vi "Webcam_Image2String.vi"(7 "file (use dialog)":path=path "/home/pi/temp.jpg", 8 "error in (no error)":errorcluster, 10 "imagegray":u8[][](array[numeric]), 11 "Image Pixels":u32[][](array[numeric])) -> (0 "error out":errorcluster, 3 "string":string)   [LabVIEW 2014, in "QwaveSys RPi Training Library.lvlib"]
uses:
  <vilib>/Q-Wave Systems/QwaveSys RPi Training Package (Demo)/Addons/QwaveSys RPi Training Library.lvlib
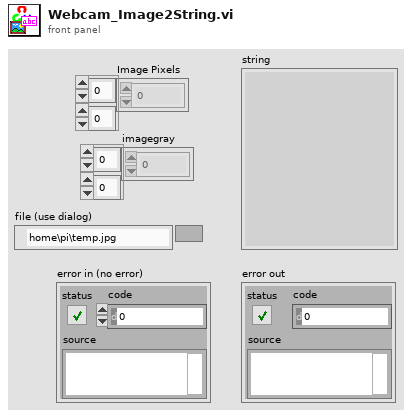
[diagram p1: front panel]
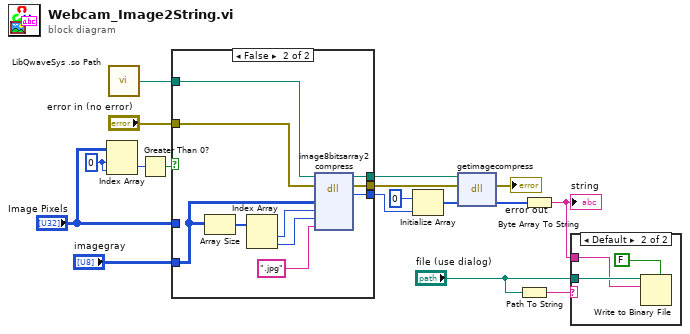
[diagram p0: block diagram]
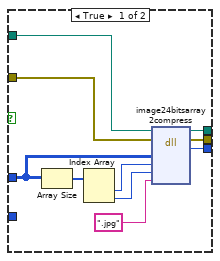
[diagram p2: hidden frame]
diagram:
  w6 = 0 ("index (row)")
  n1 = Index Array(array="Image Pixels", index (row)=w6, index (col)=w6) -> (element=w4:u32)
  n2 = call <vilib>:"LibQwaveSys .so Path.vi"() -> ("Lib QwaveSys .so Path"=w3:path)  [unwired: 5 in]
  n3 = Greater Than 0?(x=w4) -> (x > 0?=w5:bool)
  n4 = case shown="False" w5 {
    tunnel: [w27 w37] -> w15
    tunnel: [w26 w36] -> w14
    tunnel: "Image Pixels" -> [w21 _]
    tunnel: "imagegray" -> [_ w31]
    tunnel: w3 -> [w20 w30]
    tunnel: "error in (no error)" -> [w18 w29]
    tunnel: [w19 w28] -> w1
    frame True {
      n5 = Array Size(array=w21) -> (size(s)=w25:i32[])
      n6 = Index Array(array=w25) -> (element #1=w22:i32, element #2=w23:i32)  [unwired: 2 in]
      n7 = dll-call lib="libqwavesys.so" fn="image24bitsarray2compress"(path in=w20, error in=w18, "img"=w21, "cols"=w22, "rows"=w23, "file_extension"=".jpg") -> (path out=w19:path, error out=w27:errorcluster, "return type"=w26:i32)  [unwired: 5 in]
    }
    frame False {
      n8 = Array Size(array=w31) -> (size(s)=w35:i32[])
      n9 = Index Array(array=w35) -> (element #1=w32:i32, element #2=w33:i32)  [unwired: 2 in]
      n10 = dll-call lib="libqwavesys.so" fn="image8bitsarray2compress"(path in=w30, error in=w29, "img"=w31, "cols"=w32, "rows"=w33, "file_extension"=".jpg") -> (path out=w28:path, error out=w37:errorcluster, "return type"=w36:i32)  [unwired: 5 in]
    }
  }
  n11 = Initialize Array(u8 0 ("data"), w14) -> (w12:u8[])
  n12 = dll-call lib="libqwavesys.so" fn="getimagecompress"(path in=w1, error in=w15, "data"=w12) -> (error out=→"error out":errorcluster, "data"=w16:u8[])  [unwired: 2 in, 1 out]
  n13 = Path To String(path="file (use dialog)") -> (string=w10:string)
  n14 = Byte Array To String(unsigned byte array=w16) -> (string=w13:string)
  "string" <- w13
  n15 = case shown="Default" w10 {
    tunnel: "file (use dialog)" -> [_ w39]
    tunnel: w13 -> [_ w38]
    frame "/" {
    }
    frame Default {
      n16 = Write to Binary File(file (use dialog)=w39, data=w38, 5:FALSE ("prepend array or string size? (T)")) -> ()  [unwired: 3 in, 3 out]
    }
  }
